vi "Template - Scope Acquire Multiple Waveforms.vi"() -> ()   [LabVIEW 2013]
doc: "This example shows how to configure multiple channels and acquire waveforms from multiple channels."
uses:
  <instrlib>/_Template - Scope/Public/Data/Read Waveform (Multiple).vi
  <instrlib>/_Template - Scope/Template - Scope.lvlib
panel:
  in  "Maximum Time (10000 ms)":u32=10000
  in  "Serial Configuration":T1={"Baud Rate"=9600, "Parity"=0, "Data Bits"=7, "Stop Bits"=10, "Flow Control"=0} {"Flow Control" items=["None", "XON/XOFF", "RTS/CTS", "XON/XOFF & RTS/CTS", "DTR/DSR", "XON/XOFF & DTR/DSR"]; "Stop Bits" items=["1.0"=10, "1.5"=15, "2.0"=20]; "Data Bits" items=["7"=7, "8"=8]; "Parity" items=["None", "Odd", "Even", "Mark", "Space"]; "Baud Rate" items=["300"=300, "600"=600, "1200"=1200, "2400"=2400, "4800"=4800, "9600"=9600, "19200"=19200]}
  in  "Probe Attenuation (1.0)":dbl=1.0
  in  "Vertical Coupling (1: DC)":u16(ring)=1 items=["AC", "DC", "Ground"]
  in  "Channel (2: Channel 2)":u16(ring)=2 items=["Channel 1"=1, "Channel 2"=2]
  in  "Probe Attenuation (10.0)":dbl=10.0
  in  "Vertical Coupling (1: DC)":u16(ring)=1 items=["AC", "DC", "Ground"]
  in  "Channel (1: Channel 1)":u16(ring)=1 items=["Channel 1"=1, "Channel 2"=2]
  out "Waveform Data":waveform(dbl)[](graph)
  in  "VISA resource name":refnum<visa-resource-name>
  # "(c) 2007 <Enter Company Name Here>.  ALL RIGHTS RESERVED."
  # "Channel A"
  # "Channel B"
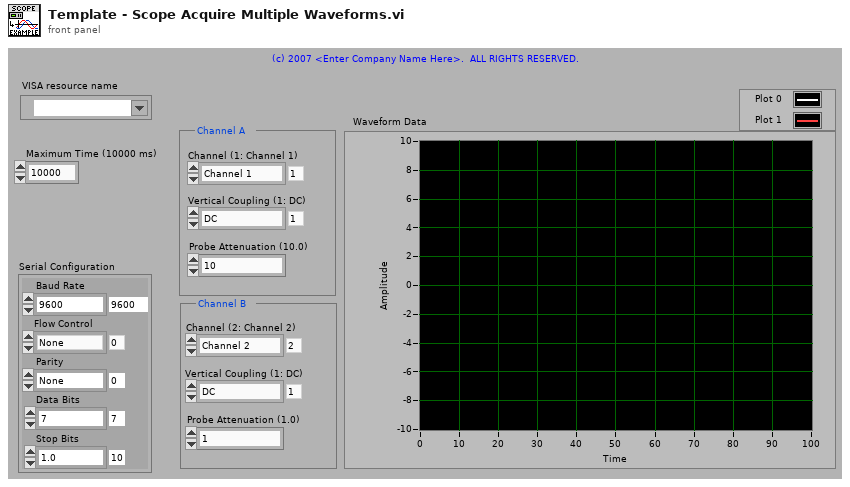
[diagram p1: front panel]
types:
  T1 = cluster{"Baud Rate":u32, "Parity":u16, "Data Bits":u16, "Stop Bits":u16, "Flow Control":u16}
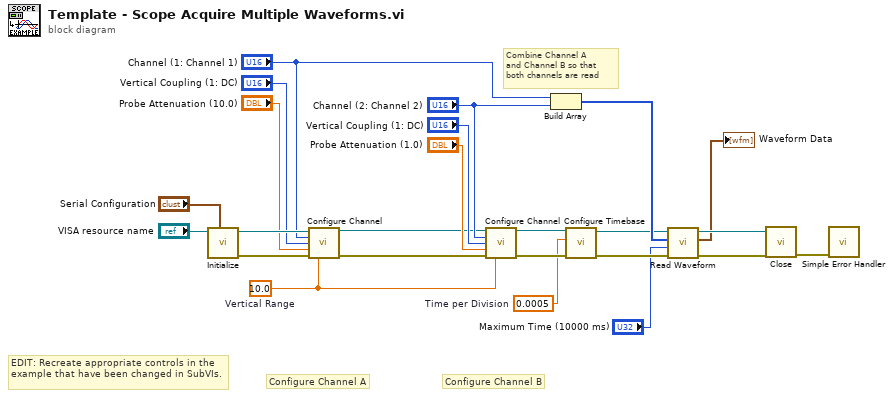
[diagram p0: block diagram]
diagram:
  w8 = 0.0005  # Time per Division
  w14 = 10.0  # Vertical Range
  # "EDIT: Recreate appropriate controls in the example that have been changed in SubVIs."
  # "Combine Channel A\nand Channel B so that\nboth channels are read"
  # "Configure Channel B"
  # "Configure Channel A"
  n1 = call <instrlib>:"Initialize.vi"("Serial Configuration"="Serial Configuration", "VISA resource name"="VISA resource name") -> ("error out"=w21:errorcluster, "VISA resource name out"=w22:refnum<visa-resource-name>)  [unwired: 8 in]
  n2 = call <instrlib>:"Configure Channel.vi"("VISA resource name"=w22, "Channel (1: Channel 1)"="Channel (1: Channel 1)", "Vertical Coupling (1: DC)"="Vertical Coupling (1: DC)", "Probe Attenuation (1.0)"="Probe Attenuation (10.0)", "error in (no error)"=w21, "Vertical Range (10.0 V)"=w14) -> ("VISA resource name out"=w10:refnum<visa-resource-name>, "error out"=w9:errorcluster)  [unwired: 8 in]
  n3 = call <instrlib>:"Configure Channel.vi"("VISA resource name"=w10, "Channel (1: Channel 1)"="Channel (2: Channel 2)", "Vertical Coupling (1: DC)"="Vertical Coupling (1: DC)", "Probe Attenuation (1.0)"="Probe Attenuation (1.0)", "error in (no error)"=w9, "Vertical Range (10.0 V)"=w14) -> ("VISA resource name out"=w20:refnum<visa-resource-name>, "error out"=w19:errorcluster)  [unwired: 8 in]
  n4 = Build Array("Channel (1: Channel 1)", "Channel (2: Channel 2)") -> (w2:u16[])
  n5 = call <instrlib>:"Configure Timebase.vi"("error in (no error)"=w19, "Time per Division (0.0005 s)"=w8, "VISA resource name"=w20) -> ("error out"=w4:errorcluster, "VISA resource name out"=w1:refnum<visa-resource-name>)  [unwired: 7 in]
  n6 = call-poly <instrlib>:"Read Waveform.vi"("error in (no error)"=w4, "Maximum Time (10000 ms)"="Maximum Time (10000 ms)", "Channels"=w2, "VISA resource name"=w1) -> ("error out"=w5:errorcluster, "Waveform Data"=→"Waveform Data":waveform(dbl)[], "VISA resource name out"=w7:refnum<visa-resource-name>)  [unwired: 5 in]
  n7 = call <instrlib>:"Close.vi"("error in (no error)"=w5, "VISA resource name"=w7) -> ("error out"=w23:errorcluster)  [unwired: 9 in]
  n8 = call <vilib>:"Simple Error Handler.vi"("error in (no error)"=w23) -> ()  [unwired: 4 in, 5 out]
